vi "Test 1.vi"(8 "error in (no error)":errorcluster, 11 "Test Case In":refnum<class "Tests.lvclass">) -> (0 "error out":errorcluster, 3 "Test Case Out":refnum<class "Tests.lvclass">)   [LabVIEW 2021, in "Tests.lvclass"]
uses:
  Tests.lvclass
  C:/Program Files (x86)/National Instruments/LabVIEW 2021/vi.lib/Astemes/LUnit/Test Case.lvclass
  <vilib>/Astemes/LUnit/Test Case.lvclass/Test Case.ctl
  4993e8ee-a06a-463a-9684-69129f64d5ce.vi
  <vilib>/Astemes/LUnit/Append Pass Result.vi
  <vilib>/Astemes/LUnit/Append Fail Result.vi
  <vilib>/Astemes/LUnit/Compare Variants.vi
  <vilib>/Astemes/LUnit/Describe Comparison of Arrays.vi
  <vilib>/Astemes/LUnit/Variant to string.vi
  <vilib>/AdvancedString/1D String Array to Delimited String.vi
  <vilib>/Utility/Data Type/Get Type Information.vi
  <vilib>/Utility/LVClass/Get LV Class Name.vi
  Tests.lvclass/Tests.ctl
  Proto/Instruction.lvclass
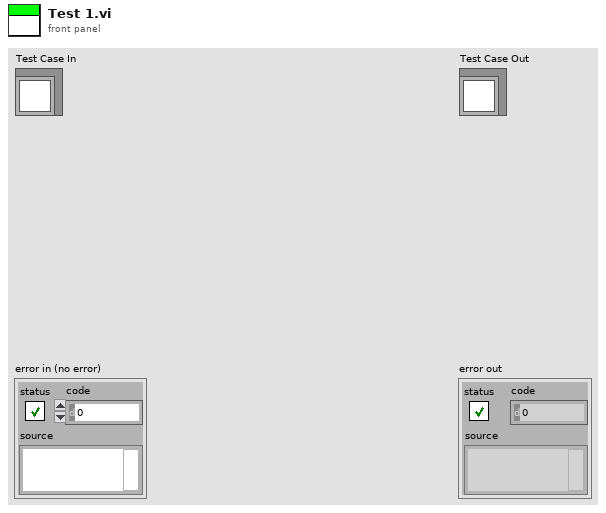
[diagram p1: front panel]
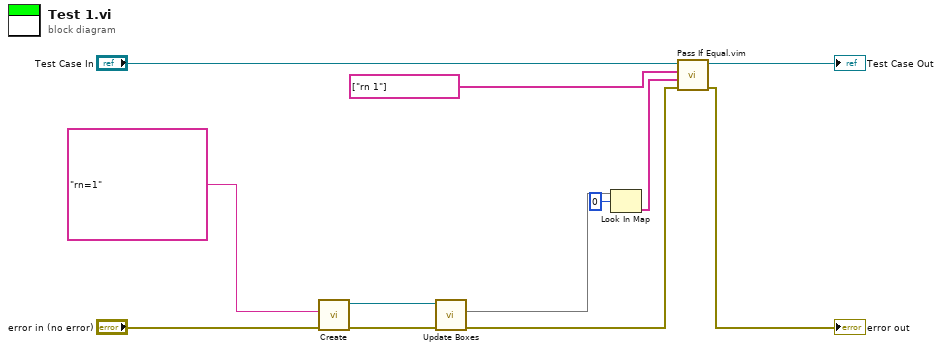
[diagram p0: block diagram]
diagram:
  n1 = call "Create.vi"("error in (no error)"="error in (no error)", "Input"="rn=1") -> ("error out"=w8:errorcluster, "Proto"=w6:refnum<class "Instruction.lvclass">)  [unwired: 8 in]
  n2 = call "Update Boxes.vi"("error in (no error)"=w8, "Instruction In"=w6) -> ("error out"=w7:errorcluster, "Boxes out"=w4:map{i32, string[]})  [unwired: 7 in, 1 out]
  n3 = Look In Map(map=w4, key=0) -> (value=w2:string[])  [unwired: 1 in, 1 out]
  n4 = call "Pass If Equal.vim"("error in (no error)"=w7, "Actual"=w2, "Expected"=string[] ["rn 1"] ("value"), "LUnit Test Case In"="Test Case In") -> ("error out"=→"error out":errorcluster, "LUnit Test Case Out"=→"Test Case Out":refnum<class "Tests.lvclass">)  [unwired: 6 in]
